vi "Actor Core.vi"(8 "error in":errorcluster, 11 "NI_DAQmx(AI) in":refnum<class "NI_DAQmx(AI).lvclass">) -> (0 "error out":errorcluster, 3 "Actor out":refnum<class "Actor.lvclass">)   [LabVIEW 2025, in "NI_DAQmx(AI).lvclass"]
doc: "<p>(<strong>Filename</strong>: <span class=\"dnl\">Actor Framework.lvlib:Actor.lvclass:Actor Core.vi</span>)</p>\n<p>Receives messages to the actor, reacts to them, and initiates any error handling that may shut the actor down.</p>\n<p>Descendant classes may override this VI to append parallel tasks for the actor to complete while it handles messages. Overrides use the <a href=\"nihelplauncher://docs/csh?context=lvcore_glang_udclass\">Call Parent Class Method</a> node.</p>"
uses:
  NI_DAQmx(AI).lvclass
  <vilib>/ActorFramework/Actor/Actor.lvclass
  NI_DAQmx(AI).lvclass/NI_DAQmx(AI).ctl
  DAQ_Abstr/Task_Type/AI_Task/AI_Task/AI_Task.lvclass
panel:
  out "Waveform Graph":waveform(dbl)[](graph)
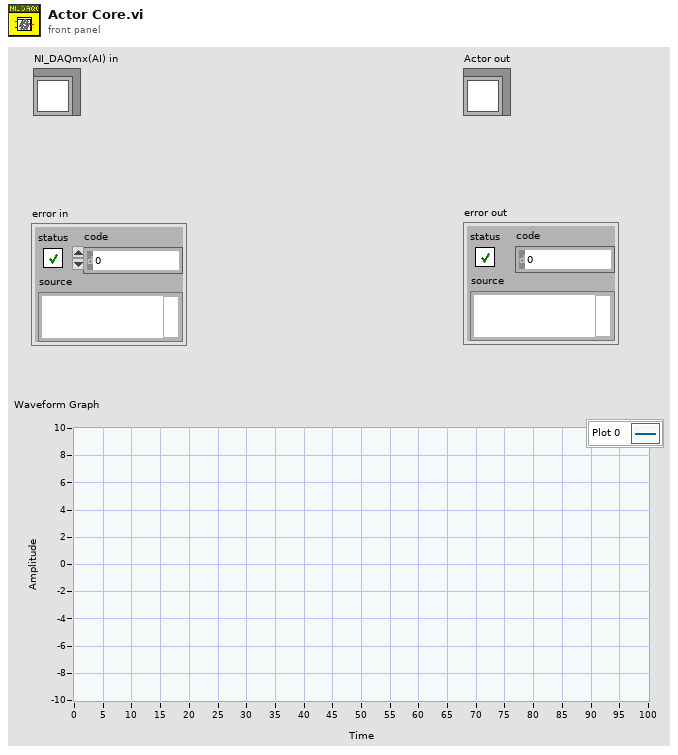
[diagram p1: front panel]
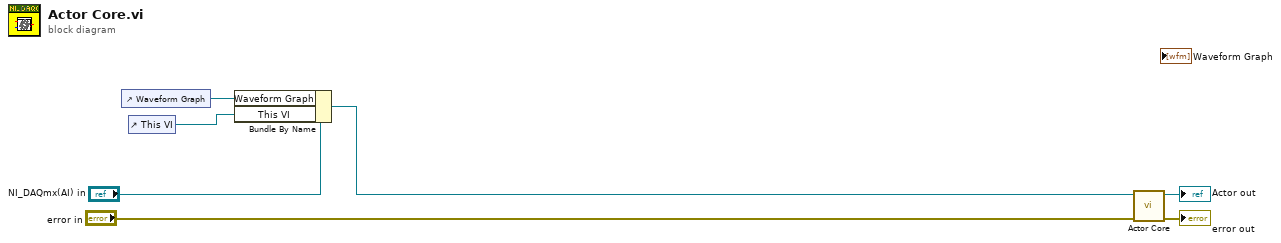
[diagram p0: block diagram]
diagram:
  n1 = control-ref of="Waveform Graph"() -> (w3:refnum<vi>)
  n2 = control-ref of="This VI"() -> (w1:refnum<vi>)
  n3 = Bundle By Name(cluster="NI_DAQmx(AI) in", "Waveform Graph"=w3, "This VI"=w1) -> (w2:refnum<class "NI_DAQmx(AI).lvclass">)
  n4 = call-parent "Actor Core.vi"("error in"="error in", "Actor in"=w2) -> ("error out"=→"error out":errorcluster, "Actor out"=→"Actor out":refnum<class "Actor.lvclass">)  [unwired: 8 in]
